vi "Encoder_Read_sub_VI.vi"() -> ()   [LabVIEW 2017]
uses:
  <vilib>/myRIO/Express VI/Onboard IO/Encoder/Encoder Express VI.xnode
  <vilib>/myRIO/Instrument Drivers/Onboard IO/Encoder/vis/Read.vi
  <vilib>/myRIO/Instrument Drivers/Onboard IO/Encoder/Encoder.lvlib
  <vilib>/myRIO/Common/Instrument Driver Framework/myRIO v1.0/Encoder/typedefs/Encoder Signal Mode.ctl
  <vilib>/myRIO/Common/Instrument Driver Framework/myRIO v1.0/Encoder/typedefs/Encoder Channels Enum.ctl
  <vilib>/myRIO/Common/Instrument Driver Framework/Utilities/typedefs/Generic FPGA Reference.ctl
  <vilib>/myRIO/Common/Instrument Driver Framework/Utilities/typedefs/myRIO v1.0 Reference.ctl
  <vilib>/myRIO/Common/Instrument Driver Framework/Utilities/typedefs/Hardware Version Enum.ctl
  <vilib>/myRIO/Common/Instrument Driver Framework/Utilities/typedefs/myRIO Generic Hardware Reference.ctl
  <vilib>/myRIO/Instrument Drivers/Onboard IO/Encoder/typedefs/Encoder Reference.ctl
  <vilib>/myRIO/Instrument Drivers/Onboard IO/Encoder/vis/myRIO Encoder Open.xnode
  <vilib>/myRIO/Common/Instrument Driver Framework/Utilities/vis/Is FPGA Ref Available.vi
  <vilib>/myRIO/Common/Instrument Driver Framework/myRIO v1.0/Encoder/vis/myRIO v1.1 Open Encoder.vi
  <vilib>/myRIO/Common/Instrument Driver Framework/myRIO v1.0/Encoder/vis/myRIO v1.0 Configure Encoder.vi
  <vilib>/myRIO/Common/Instrument Driver Framework/myRIO v1.0/Encoder/typedefs/Encoder Configuration v1.0.ctl
  <vilib>/userdefined/High Color/nirio_resource_hc.ctl
  <vilib>/myRIO/Common/Instrument Driver Framework/myRIO v1.0/Encoder/typedefs/Encoder Count Direction Enum.ctl
panel:
  out "X-axis direction":enum16{"Counting Up", "Counting Down"}(ring)
  out "Y-axis direction":enum16{"Counting Up", "Counting Down"}(ring)
  out "Encoder Output":T1
  in  "Encoder Input":T1
  out "error out":errorcluster
  in  "error in (no error)":errorcluster
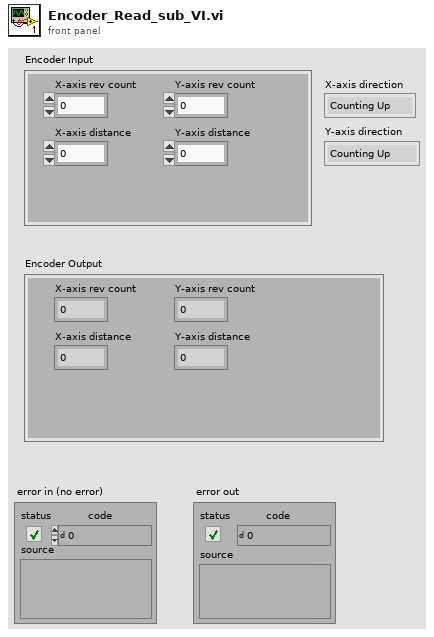
[diagram p1: front panel]
types:
  T1 = cluster{"Y-axis rev count":i32, "Y-axis distance":dbl, "X-axis rev count":i32, "X-axis distance":dbl}
  T2 = typedef "Encoder Count Direction Enum.ctl" = enum16{"Counting Up", "Counting Down"}
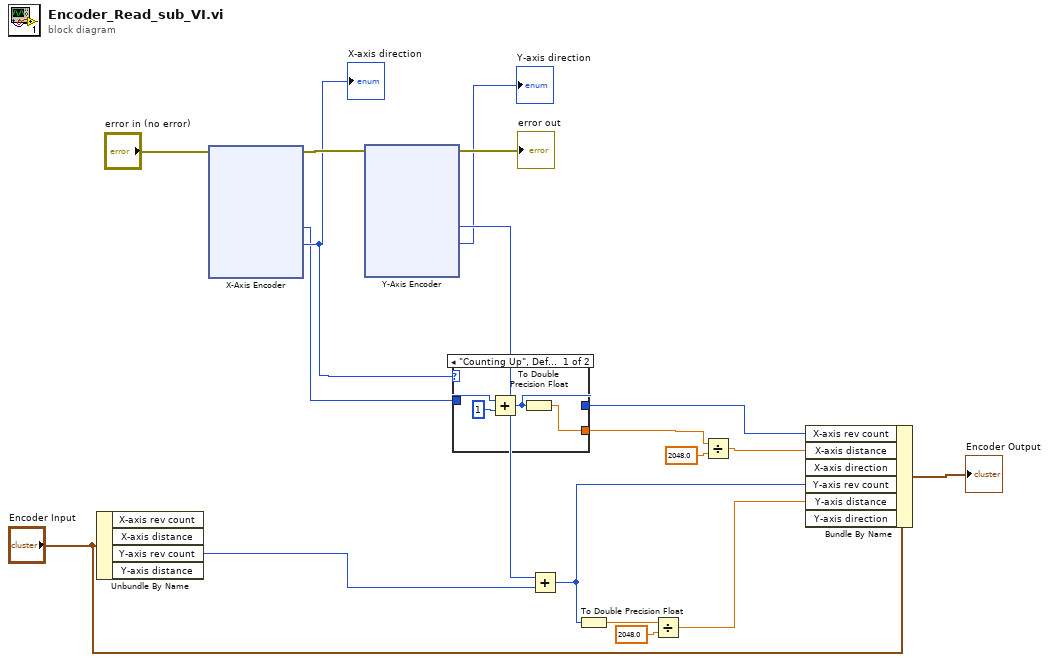
[diagram p0: block diagram]
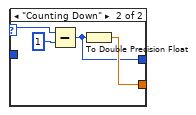
[diagram p2: hidden frame]
diagram:
  n1 = Unbundle By Name("Encoder Input") -> ("Y-axis rev count"=w11:i32)  [unwired: 3 out]
  n2 = xnode "X-Axis Encoder"("error in (no error)"="error in (no error)") -> ("Counter Value"=w3:i32, "Counter Direction"=w4:T2, "error out"=w13:errorcluster)  [unwired: 1 in, 1 out]
  "X-axis direction" <- w4
  n3 = xnode "Y-Axis Encoder"("error in (no error)"=w13) -> ("Counter Value"=w10:i32, "Counter Direction"=→"Y-axis direction":enum16{"Counting Up", "Counting Down"}, "error out"=→"error out":errorcluster)  [unwired: 1 in, 1 out]
  n4 = case shown="\"Counting Up\", Default" w4 {
    tunnel: w3 -> [w22 w26]
    tunnel: [w21 w24] -> w2
    tunnel: [w20 w23] -> w1
    frame "Counting Up", Default {
      n5 = Add(x=w22, y=1) -> (x+y=w20:i32)
      n6 = To Double Precision Float(number=w20) -> (double precision float=w21:dbl)
    }
    frame "Counting Down" {
      n7 = Subtract(x=w26, y=1) -> (x-y=w23:i32)
      n8 = To Double Precision Float(number=w23) -> (double precision float=w24:dbl)
    }
  }
  n9 = Add(x=w10, y=w11) -> (x+y=w6:i32)
  n10 = To Double Precision Float(number=w6) -> (double precision float=w9:dbl)
  n11 = Divide(x=w9, y=2048.0) -> (x/y=w7:dbl)
  n12 = Divide(x=w2, y=2048.0) -> (x/y=w16:dbl)
  n13 = Bundle By Name(cluster="Encoder Input", "X-axis rev count"=w1, "X-axis distance"=w16, "Y-axis rev count"=w6, "Y-axis distance"=w7) -> (→"Encoder Output":T1)  [unwired: 2 in]
